vi "Read Data.vi"(8 "error in":errorcluster, 11 "Orient3d in":refnum<class "Orient3d Class.lvclass">) -> (0 "error out":errorcluster, 2 "Quaternion":T1, 3 "Orient3d out":refnum<class "Orient3d Class.lvclass">)   [LabVIEW 2011, in "Orient3d Class.lvclass"]
uses:
  Orient3d Class.lvclass
  Type Definitions/Quaternion.ctl
  Orient3d Class.lvclass/Orient3d Class.ctl
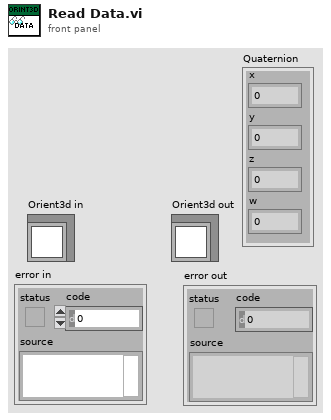
[diagram p1: front panel]
types:
  T1 = typedef "Quaternion.ctl" = cluster{"x":dbl, "y":dbl, "z":dbl, "w":dbl}
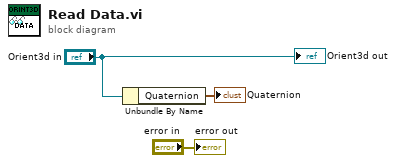
[diagram p0: block diagram]
diagram:
  n1 = Unbundle By Name("Orient3d in") -> ("Quaternion"=→"Quaternion":T1)
  "error out" <- "error in"
  "Orient3d out" <- "Orient3d in"
